vi "RichToFlatrfcontrol_KPIData.vi"(5 "OutputClusterType":T1, 11 "InputCluster":T3) -> (3 "OutputCluster":T1)   [LabVIEW 2024, in "FlexCompute_grpc_client.lvlib"]
uses:
  rfcontrol_KPIData.ctl
  rfcontrol_Status.ctl
  rfcontrol_KPIData_Flat.ctl
  FlexCompute_grpc_client.lvlib
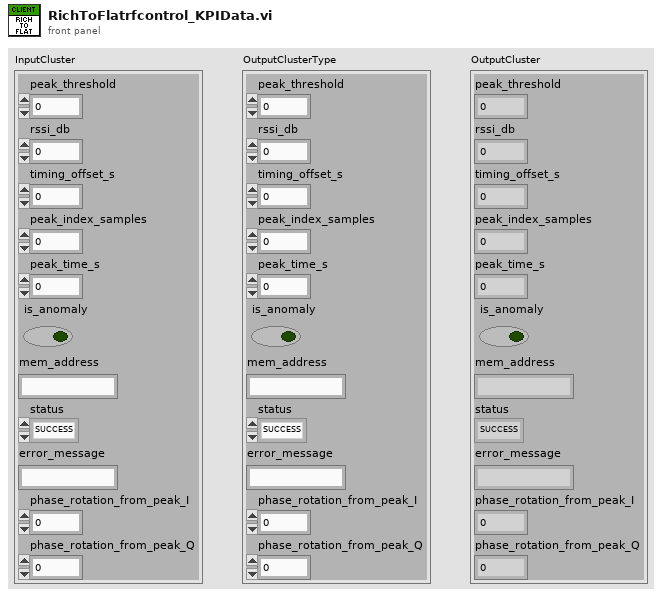
[diagram p1: front panel]
types:
  T1 = typedef "FlexCompute_grpc_client.lvlib/rfcontrol_KPIData_Flat.ctl" = cluster{"peak_threshold":dbl, "rssi_db":dbl, "timing_offset_s":dbl, "peak_index_samples":i32, "peak_time_s":dbl, "is_anomaly":bool, "mem_address":string, "status":T2, "error_message":string, "phase_rotation_from_peak_I":sgl, "phase_rotation_from_peak_Q":sgl}
  T2 = typedef "FlexCompute_grpc_client.lvlib/rfcontrol_Status.ctl" = enum32{"SUCCESS", "ERROR"}
  T3 = typedef "FlexCompute_grpc_client.lvlib/rfcontrol_KPIData.ctl" = cluster{"peak_threshold":dbl, "rssi_db":dbl, "timing_offset_s":dbl, "peak_index_samples":i32, "peak_time_s":dbl, "is_anomaly":bool, "mem_address":string, "status":T2, "error_message":string, "phase_rotation_from_peak_I":sgl, "phase_rotation_from_peak_Q":sgl}
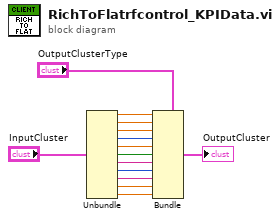
[diagram p0: block diagram]
diagram:
  n1 = Unbundle "Unbundle"("InputCluster") -> ("peak_threshold"=w11:dbl, "rssi_db"=w10:dbl, "timing_offset_s"=w9:dbl, "peak_index_samples"=w8:i32, "peak_time_s"=w7:dbl, "is_anomaly"=w6:bool, "mem_address"=w5:string, "status"=w4:T2, "error_message"=w3:string, "phase_rotation_from_peak_I"=w2:sgl, "phase_rotation_from_peak_Q"=w1:sgl)
  n2 = Bundle "Bundle"(cluster="OutputClusterType", "peak_threshold"=w11, "rssi_db"=w10, "timing_offset_s"=w9, "peak_index_samples"=w8, "peak_time_s"=w7, "is_anomaly"=w6, "mem_address"=w5, "status"=w4, "error_message"=w3, "phase_rotation_from_peak_I"=w2, "phase_rotation_from_peak_Q"=w1) -> (→"OutputCluster":T1)
